vi "alignment_main.vi"() -> ()   [LabVIEW 2011]
uses:
  global_vars.vi
  <vilib>/vision/driver/NI_Vision_Acquisition_Software.lvlib
  C:/Program Files/National Instruments/LabVIEW 2011/resource/objmgr/imaqdx.rc
panel:
  in  "stream_overlay":bool
  in  "save":bool
  in  "File Path":path
  in  "ValueDBL":dbl(slide)=1e-10 min=1e-10 max=1.0 scale=0.0..0.25
  out "Image":T1(plugin-control)
  in  "flip direction":bool
  in  "stream_OL_center_radius":dbl
  in  "stream_OL_#rings":i32
  in  "df_intial phase shift":dbl
  in  "df_#fringes":dbl=4.0 caption="#fringes"
  in  "fringe_OL_#rings":i32=20
  in  "fringe_OL_center_radius":dbl
  in  "fringe_OL_color":u32(colorbox)=16448250
  in  "b_align":bool=TRUE
  in  "b_preview fringes":bool
  in  "fullscreen?":bool
  in  "y height(Px)":i32=500
  in  "x Width(Px)":i32=1000
  in  "to second \nscreen?":bool
  in  "floating":bool=TRUE
  in  "title bar":bool=TRUE
  in  "stream_OL_color":u32(colorbox)=16448250
  in  "Close":bool
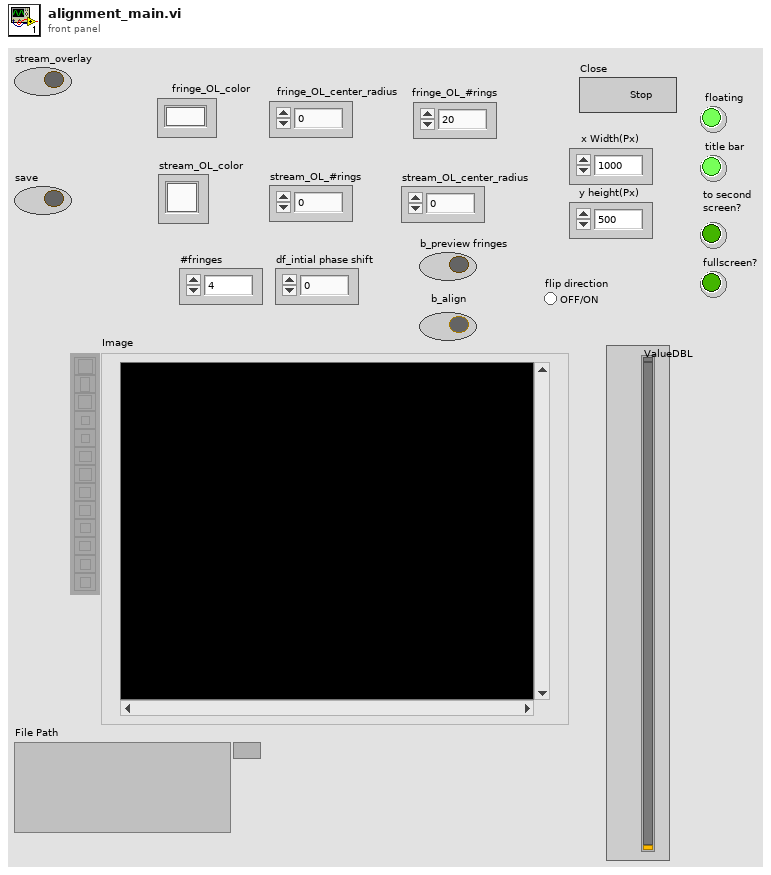
[diagram p1: front panel]
types:
  T1 = typedef "IMAQ Image.ctl" = refnum<image>
  T2 = typedef "IMAQdx.ctl" = refnum<k21>
  T3 = cluster{"Numeric Control":i16, "Numeric Control":i16}
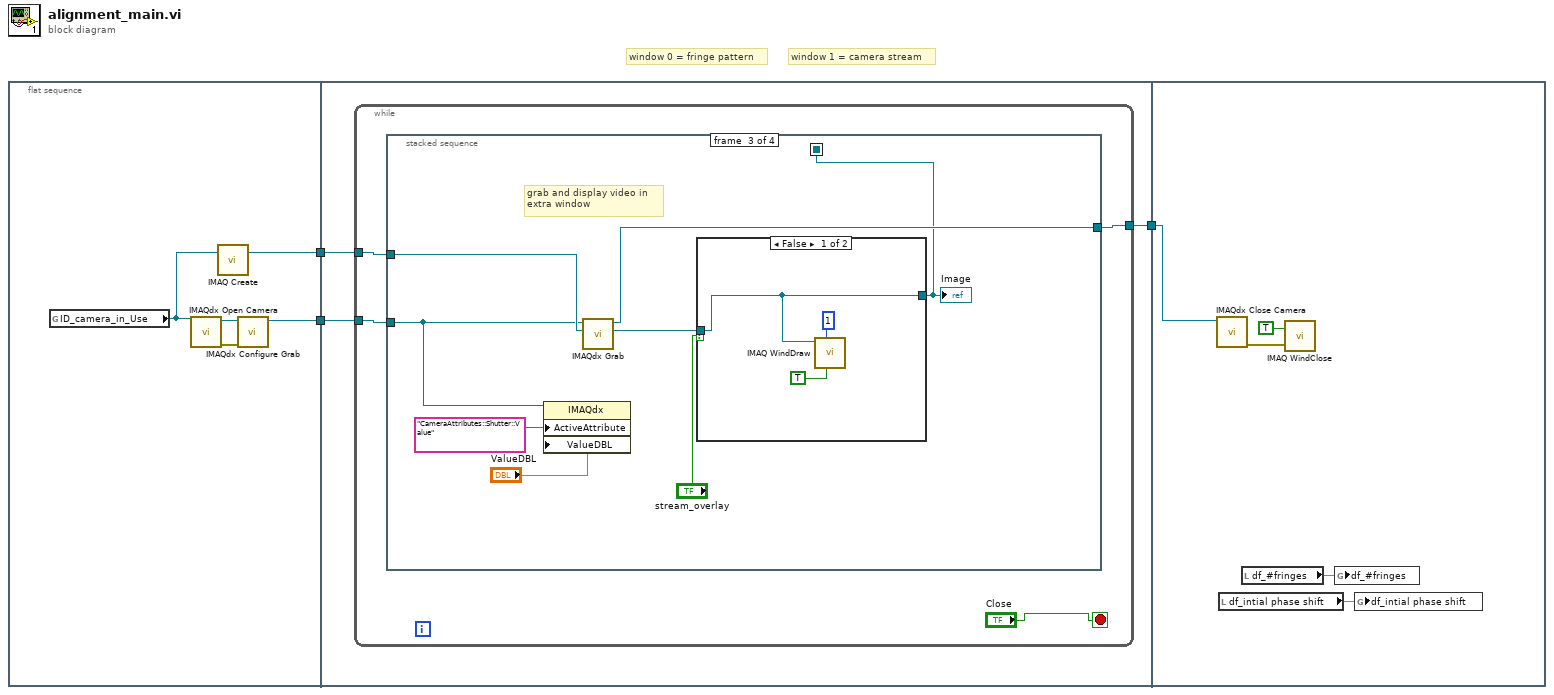
[diagram p0: block diagram]
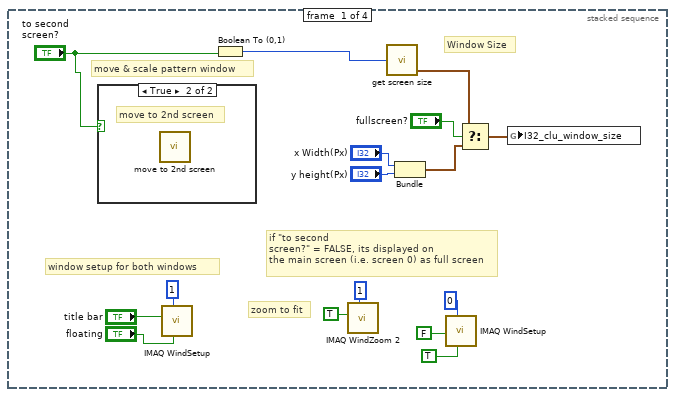
[diagram p2: hidden frame]
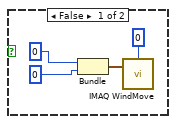
[diagram p3: hidden frame]
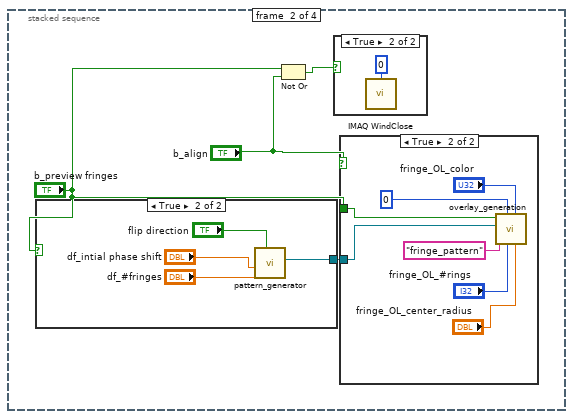
[diagram p4: hidden frame]
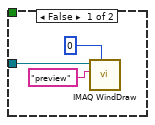
[diagram p6: hidden frame]
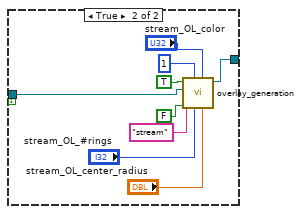
[diagram p8: hidden frame]
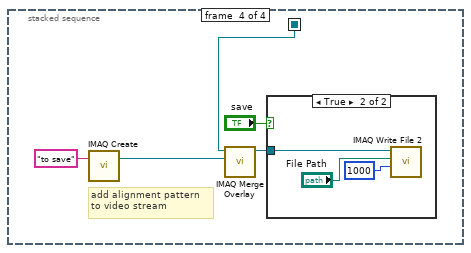
[diagram p9: hidden frame]
diagram:
  # "window 1 = camera stream"
  # "window 0 = fringe pattern"
  n1 = flat-sequence {
    tunnel: [w4] -> w2
    tunnel: [w5] -> w1
    tunnel: [w9] -> w3
    tunnel: w2 -> [w11]
    tunnel: w1 -> [w10]
    tunnel: w3 -> [w83]
    frame #0 {
      n2 = global read "global_vars.vi" "ID_camera_in_Use"() -> (w8:T2)
      n3 = call <vilib>:"IMAQdx Open Camera.vi"("Session In"=w8) -> ("error out"=w6:errorcluster, "Session Out"=w7:T2)  [unwired: 2 in, 7 out]
      n4 = call "IMAQ Create"("Image Name"=w8) -> ("New Image"=w4:T1)  [unwired: 3 in, 2 out]
      n5 = call <vilib>:"IMAQdx Configure Grab.vi"("error in"=w6, "Session In"=w7) -> ("Session Out"=w5:T2)  [unwired: 9 out]
    }
    frame #1 {
      n6 = while {
        tunnel: w10 -> [w15]
        tunnel: w11 -> [w14]
        tunnel: [w12] -> w9
        stop <- "Close" stop-if-true
        n7 = stacked-sequence {
          seq-local: [_ _ w56 _] -> [_ _ _ w75]
          tunnel: w15 -> [_ _ w60 _]
          tunnel: w14 -> [_ _ w62 _]
          tunnel: [_ _ w61 _] -> w12
          frame #0 {
            # "zoom to fit"
            # "if \"to second \nscreen?\" = FALSE, its displayed on \nthe main screen (i.e. screen 0) as full screen"
            # "window setup for both windows"
            # "Window Size"
            # "move & scale pattern window"
            n8 = case shown="True" "to second \nscreen?" {
              frame False {
                n9 = Bundle(0, 0) -> (w35:cluster{i32, i32})  [unwired: 1 in]
                n10 = call "IMAQ WindMove"("Window Number (0...15)"=0, "Coordinates (screen)"=w35) -> ()  [unwired: 3 in, 2 out]
              }
              frame True {
                # "move to 2nd screen"
                n11 = call "move to 2nd screen.vi"() -> ()  [unwired: 12 in]
              }
            }
            n12 = call "IMAQ WindSetup"("Window is floating? (No)"="floating", "Window Number (0...15)"=1, "Window has title bar? (Yes)"="title bar") -> ()  [unwired: 8 in, 1 out]
            n13 = Boolean To (0,1)(Boolean="to second \nscreen?") -> (0, 1=w31:i16)
            n14 = call "IMAQ WindZoom 2"("Window Number (0...15)"=1, "Zoom to Fit? (False)"=TRUE) -> ()  [unwired: 6 in, 4 out]
            n15 = call "get screen size.vi"("screen"=w31) -> ("wind size (width/height)"=w30:T3)  [unwired: 2 in, 2 out]
            n16 = Bundle("x Width(Px)"="x Width(Px)", "y height(Px)"="y height(Px)") -> (w28:cluster{"x Width(Px)":i32, "y height(Px)":i32})  [unwired: 1 in]
            n17 = call "IMAQ WindSetup"("Window is floating? (No)"=TRUE, "Window Number (0...15)"=0, "Window has title bar? (Yes)"=FALSE) -> ()  [unwired: 8 in, 1 out]
            n18 = Select(t=w30, s="fullscreen?", f=w28) -> (s? t:f=w29:cluster{"x Width(Px)":i32, "y height(Px)":i32})
            n19 = global write "global_vars.vi" "I32_clu_window_size"(w29) -> ()
          }
          frame #1 {
            n20 = case shown="True" "b_preview fringes" {
              tunnel: [_ w54] -> w36
              frame False {
              }
              frame True {
                n21 = call "pattern_generator.vi"("flip direction"="flip direction", "fringe number"="df_#fringes", "phase"="df_intial phase shift") -> ("fringe pattern"=w54:T1)  [unwired: 7 in, 1 out]
              }
            }
            n22 = Not Or(1:"b_align", 2:"b_preview fringes") -> (0:w37:bool)
            n23 = case shown="True" w37 {
              frame False {
              }
              frame True {
                n24 = call "IMAQ WindClose"("Window Number (0...15)"=0) -> ()  [unwired: 5 in, 1 out]
              }
            }
            n25 = case shown="True" "b_align" {
              tunnel: w36 -> [w42 w50]
              tunnel: "b_preview fringes" -> [_ w49]
              frame False {
                n26 = call "IMAQ WindDraw"("Window Number (0...15)"=0, "Title"="preview", "Image"=w42) -> ()  [unwired: 7 in, 2 out]
              }
              frame True {
                n27 = call "overlay_generation.vi"("center radius"="fringe_OL_center_radius", "Color"="fringe_OL_color", "number of rings"="fringe_OL_#rings", "Window Number (0...15)"=0, "Title"="fringe_pattern", "Image Src"=w50, "fringe preview on"=w49) -> ()  [unwired: 4 in, 1 out]
              }
            }
          }
          frame #2 {
            # "grab and display video in \nextra window"
            n28 = property class="IMAQdx"(reference=w60, "ActiveAttribute"="CameraAttributes::Shutter::Value", "ValueDBL"="ValueDBL") -> ()  [unwired: 1 in, 2 out]
            n29 = call <vilib>:"IMAQdx Grab.vi"("Image In"=w62, "Session In"=w60) -> ("Image Out"=w57:T1, "Session Out"=w61:T2)  [unwired: 2 in, 6 out]
            n30 = case shown="False" "stream_overlay" {
              tunnel: w57 -> [w65 w67]
              tunnel: [w65 w66] -> w56
              frame False {
                n31 = call "IMAQ WindDraw"("Resize to Image Size? (Y)"=TRUE, "Window Number (0...15)"=1, "Image"=w65) -> ()  [unwired: 7 in, 2 out]
              }
              frame True {
                n32 = call "overlay_generation.vi"("center radius"="stream_OL_center_radius", "Color"="stream_OL_color", "number of rings"="stream_OL_#rings", "Window Number (0...15)"=1, "Resize to Image Size? (Y)"=FALSE, "Title"="stream", "Image Src"=w67, "fringe preview on"=TRUE) -> ("stream_overlay_out"=w66:T1)  [unwired: 3 in]
              }
            }
            "Image" <- w56
          }
          frame #3 {
            # "add alignment pattern \nto video stream"
            n33 = call "IMAQ Create"("Image Name"="to save") -> ("New Image"=w76:T1)  [unwired: 3 in, 2 out]
            n34 = call "IMAQ Merge Overlay"("Image Dst"=w76, "Image Src"=w75) -> ("Image Dst Out"=w78:T1)  [unwired: 8 in, 1 out]
            n35 = case shown="True" "save" {
              tunnel: w78 -> [_ w82]
              frame False {
              }
              frame True {
                n36 = call-poly "IMAQ Write File 2"("Image Quality"=u32 1000, "File Path"="File Path", "Image"=w82) -> ()  [unwired: 7 in, 2 out]
              }
            }
          }
        }
      }
    }
    frame #2 {
      n37 = call <vilib>:"IMAQdx Close Camera.vi"("Session In"=w83) -> ("error out"=w85:errorcluster)  [unwired: 1 in, 9 out]
      n38 = local read "df_intial phase shift"() -> (w87:dbl)
      n39 = local read "df_#fringes"() -> (w86:dbl)
      n40 = call "IMAQ WindClose"("Close All Windows (False)"=TRUE, "error in (no error)"=w85) -> ()  [unwired: 4 in, 1 out]
      n41 = global write "global_vars.vi" "df_#fringes"(w86) -> ()
      n42 = global write "global_vars.vi" "df_intial phase shift"(w87) -> ()
    }
  }
